vi "Test Welch Output.vi"() -> ()   [LabVIEW 2015]
uses:
  <vilib>/Analysis/baseanly.llb/Mean (DBL).vi
  <vilib>/addons/Time Series Analysis/Correlation and Spectral Analysis.llb/TSA Welch (Array).vi
  <vilib>/Analysis/NI_AALBase.lvlib
  <vilib>/addons/_Advanced Signal Processing/NI_AdvSigProcTSA.lvlib
panel:
  out "mean":dbl format="%.5f"
  out "df":dbl
  out "Waveform Graph":dbl[](graph)
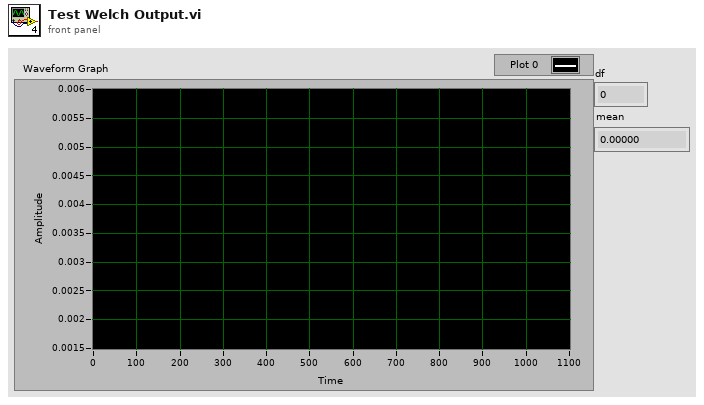
[diagram p1: front panel]
types:
  T1 = cluster{"window":u16, "length":i32, "overlap (%)":dbl}
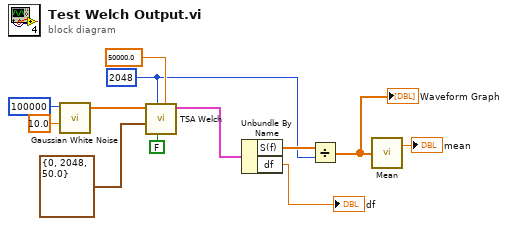
[diagram p0: block diagram]
diagram:
  w2 = 2048 ("frequency bins")
  n1 = call <vilib>:"Gaussian White Noise.vi"("standard deviation"=10.0, "samples"=100000) -> ("Gaussian noise pattern"=w10:dbl[])  [unwired: 8 in, 1 out]
  n2 = call-poly <vilib>:"TSA Welch.vi"("sampling rate"=50000.0, "dB on? (T)"=FALSE, "frequency bins"=w2, "window info"=T1 {"window"=0, "length"=2048, "overlap (%)"=50.0}, "Xt"=w10) -> ("PSD"=w6:cluster{"f0":dbl, "df":dbl, "S(f)":dbl[]})  [unwired: 5 in, 1 out]
  n3 = Unbundle By Name(w6) -> ("S(f)"=w4:dbl[], "df"=→"df":dbl)
  n4 = Divide(x=w4, y=w2) -> (x/y=w1:dbl[])
  "Waveform Graph" <- w1
  n5 = call-poly <vilib>:"Mean.vi"("X"=w1) -> ("mean"=→"mean":dbl)  [unwired: 1 out]
